vi "RequestPulse.vi"(8 "error in (no error)":errorcluster, 11 "DMC_1000B in":refnum<class "DMC_1000B.lvclass">) -> (0 "error out":errorcluster, 2 "Pulse":dbl, 3 "DMC_1000B out":refnum<class "DMC_1000B.lvclass">)   [LabVIEW 2019, in "DMC_1000B.lvclass"]
uses:
  DMC_1000B.lvclass
  LLB/DMC1000B/Dmc1000/Dmc1000.lvlib
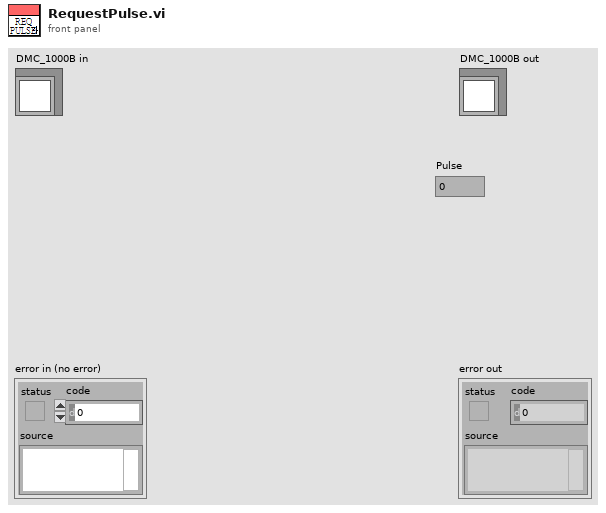
[diagram p1: front panel]
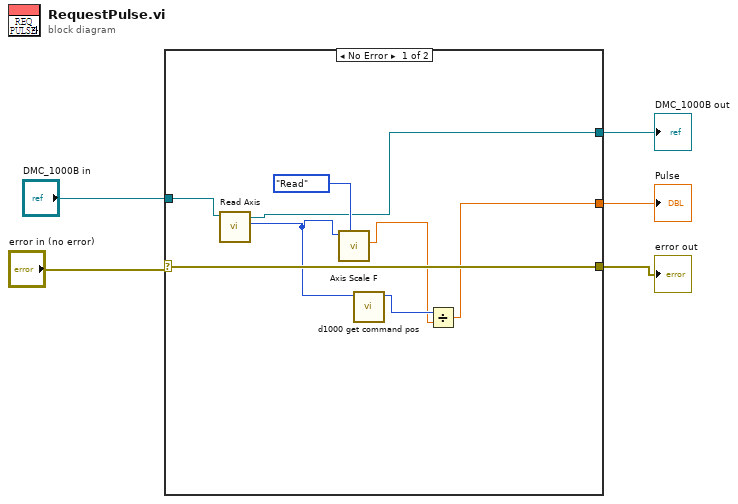
[diagram p0: block diagram]
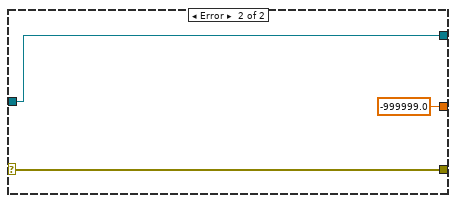
[diagram p2: hidden frame]
diagram:
  n1 = case shown="No Error" "error in (no error)" {
    selector: "error in (no error)" -> [w13 w16]
    tunnel: [w13 w16] -> w4
    tunnel: "DMC_1000B in" -> [w12 w14]
    tunnel: [w10 -999999.0] -> w2
    tunnel: [w6 w14] -> w1
    frame No Error {
      n2 = call-dynamic "Read Axis.vi"("AxisCard in"=w12) -> ("Axis"=w9:u32, "AxisCard out"=w6:refnum<class "DMC_1000B.lvclass">)  [unwired: 8 in, 1 out]
      n3 = call "Axis Scale F.vi"("Enum"=enum16{"Initial", "Read"}."Read", "Axis"=w9) -> ("Scale"=w8:dbl)  [unwired: 8 in, 1 out]
      n4 = call "d1000 get command pos.vi"("axis"=w9) -> ("function return"=w11:i32)  [unwired: 10 in]
      n5 = Divide(x=w11, y=w8) -> (x/y=w10:dbl)
    }
    frame Error {
    }
  }
  "error out" <- w4
  "DMC_1000B out" <- w1
  "Pulse" <- w2
